vi "SetReadOutRate.vi"(8 "error in (no error)":errorcluster, 11 "Camera_Prime95B in":refnum<class "Camera_Prime95B.lvclass">) -> (0 "error out":errorcluster, 3 "Camera_Prime95B out":refnum<class "Camera_Prime95B.lvclass">)   [LabVIEW 2020, in "Camera_Prime95B.lvlib" / "Camera_Prime95B.lvclass"]
uses:
  Camera_Prime95B.lvclass
  Camera_Prime95B.lvclass/Camera_Prime95B.ctl
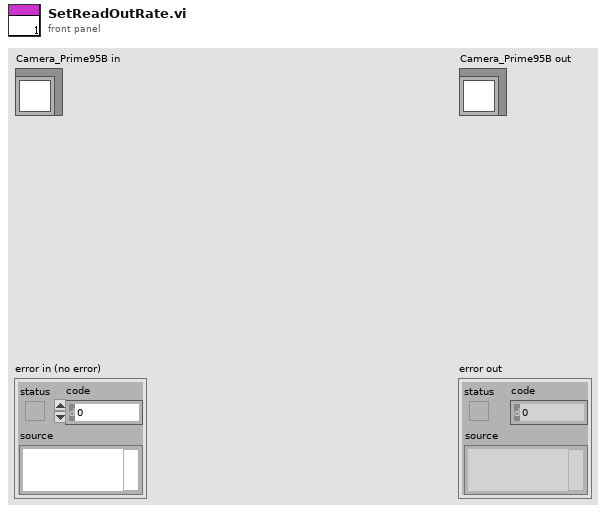
[diagram p1: front panel]
types:
  T1 = typedef "Device.lvlib/DeviceStatus.ctl" = i32
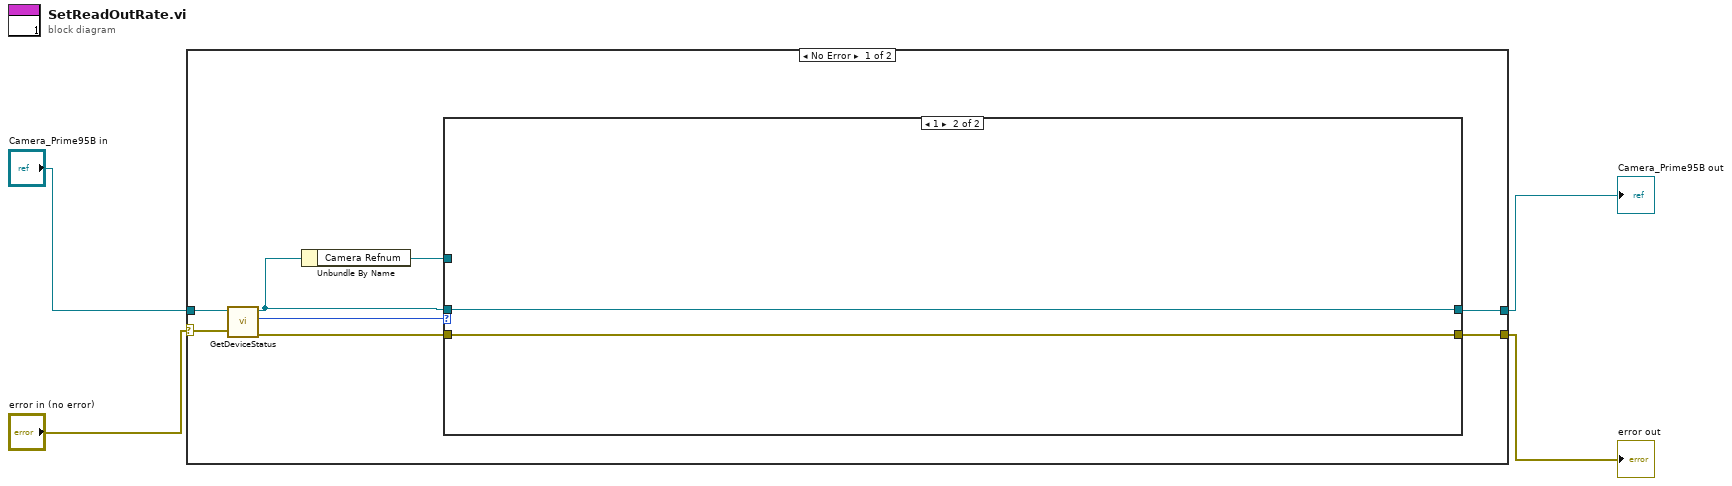
[diagram p0: block diagram]
diagram:
  n1 = case shown="No Error" "error in (no error)" {
    selector: "error in (no error)" -> [w11 w18]
    tunnel: [w12 w18] -> w3
    tunnel: [w6 w17] -> w4
    tunnel: "Camera_Prime95B in" -> [w5 w17]
    frame No Error {
      n2 = call-dynamic "GetDeviceStatus.vi"("error in (no error)"=w11, "Camera_Prime95B in"=w5) -> ("error out"=w9:errorcluster, "Status"=w10:T1, "Camera_Prime95B out"=w7:refnum<class "Camera_Prime95B.lvclass">)  [unwired: 7 in]
      n3 = Unbundle By Name(w7) -> ("Camera Refnum"=w8:refnum<k24>)
      n4 = case shown="1" w10 {
        tunnel: [w13 w16] -> w12
        tunnel: w8 -> [_ _]
        tunnel: w9 -> [w13 w16]
        tunnel: w7 -> [w14 w15]
        tunnel: [w14 w15] -> w6
        frame 0, Default {
        }
        frame 1 {
        }
      }
    }
    frame Error {
    }
  }
  "error out" <- w3
  "Camera_Prime95B out" <- w4
